vi "TCP SSH.vi"(6 "States":T1, 7 "Error In":errorcluster) -> (0 "Error  Out":errorcluster, 2 "Response":string)   [LabVIEW 2021]
uses:
  controls/TCP states.ctl
  <vilib>/Field R&D Services/LIBSSH2 for LabVIEW/Toolkit/Session/Support/Create from SSH.vi
  <vilib>/Field R&D Services/LIBSSH2 for LabVIEW/Toolkit/Session/Support/Password Authentication.vi
  <vilib>/Field R&D Services/LIBSSH2 for LabVIEW/Toolkit/Channel/Support/Create from Session.vi
  <vilib>/Field R&D Services/LIBSSH2 for LabVIEW/Toolkit/Channel/Support/Destroy to Session.vi
  <vilib>/Field R&D Services/LIBSSH2 for LabVIEW/Toolkit/Session/Support/Destroy to SSH.vi
  <vilib>/Field R&D Services/LIBSSH2 for LabVIEW/Toolkit/Channel/Channel.lvclass
  <vilib>/Field R&D Services/LIBSSH2 for LabVIEW/Toolkit/SSH/SSH.lvclass
  <vilib>/Field R&D Services/LIBSSH2 for LabVIEW/Toolkit/Session/Session.lvclass
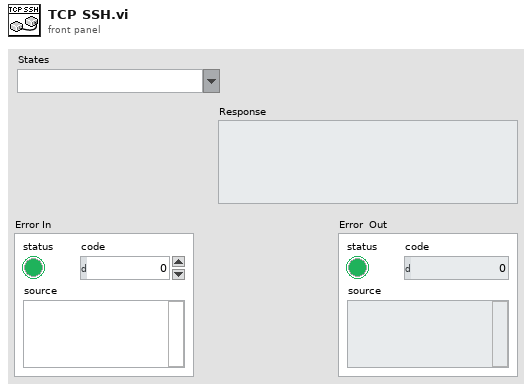
[diagram p1: front panel]
types:
  T1 = typedef "TCP states.ctl" = string
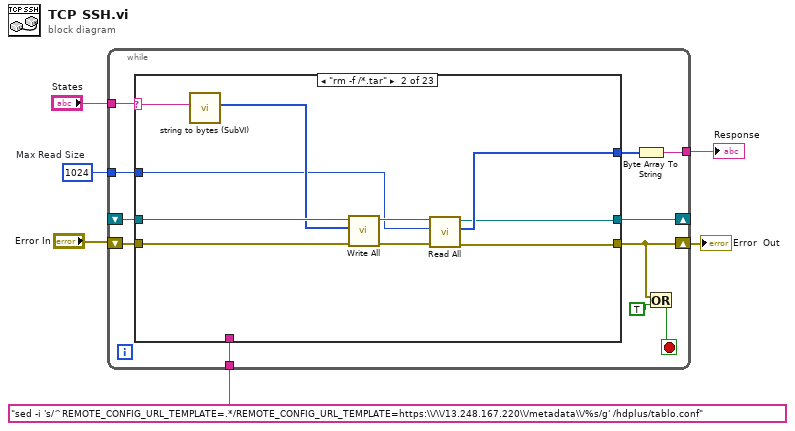
[diagram p0: block diagram]
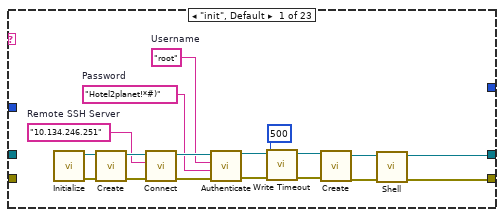
[diagram p2: hidden frame]
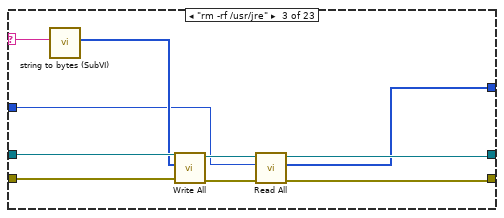
[diagram p3: hidden frame]
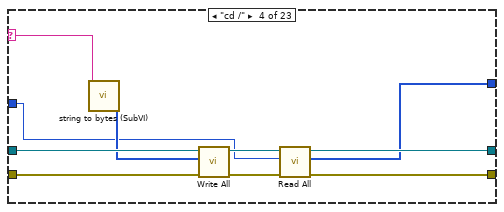
[diagram p4: hidden frame]
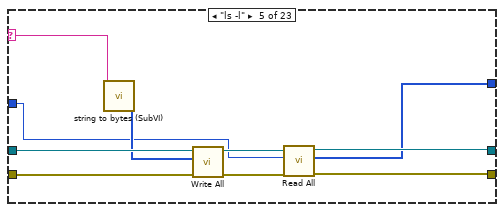
[diagram p5: hidden frame]
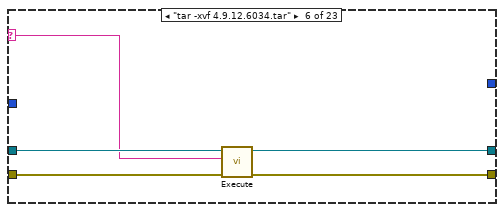
[diagram p6: hidden frame]
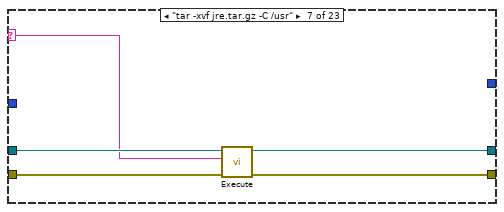
[diagram p7: hidden frame]
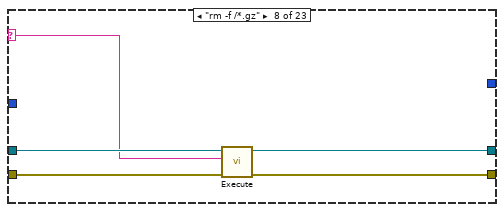
[diagram p8: hidden frame]
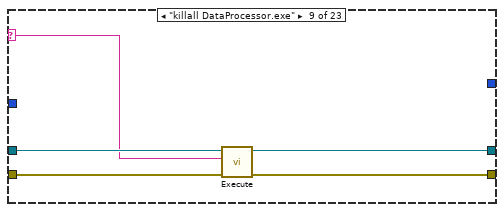
[diagram p9: hidden frame]
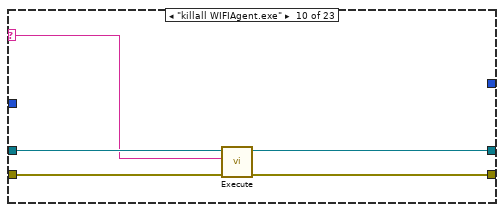
[diagram p10: hidden frame]
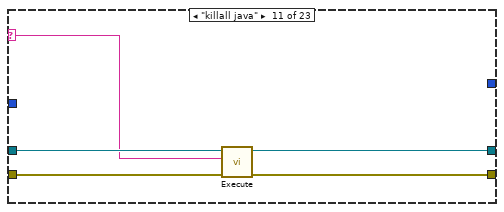
[diagram p11: hidden frame]
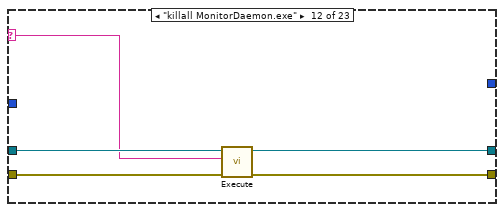
[diagram p12: hidden frame]
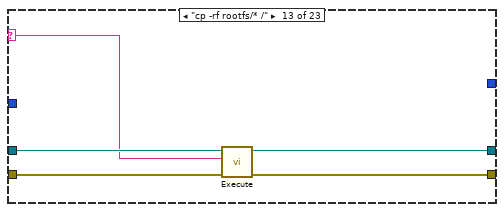
[diagram p13: hidden frame]
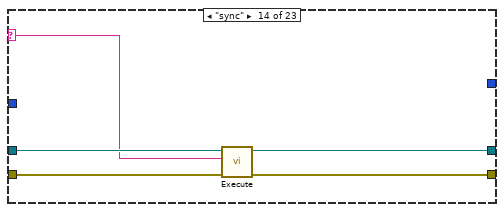
[diagram p14: hidden frame]
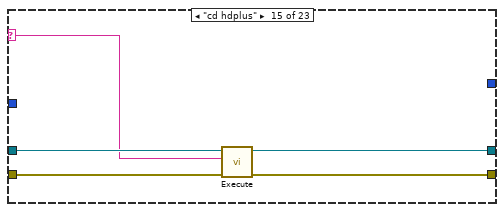
[diagram p15: hidden frame]
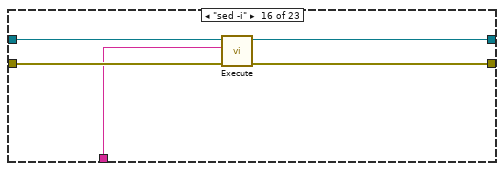
[diagram p16: hidden frame]
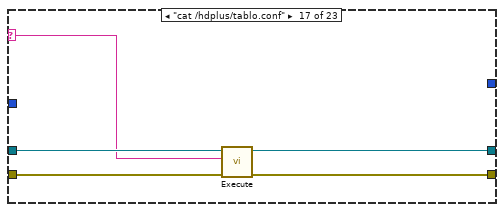
[diagram p17: hidden frame]
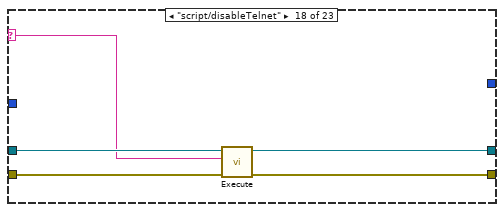
[diagram p18: hidden frame]
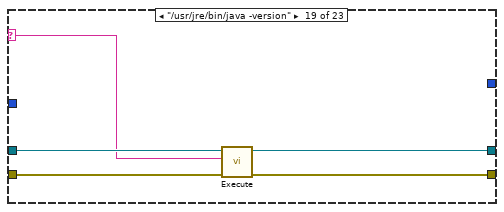
[diagram p19: hidden frame]
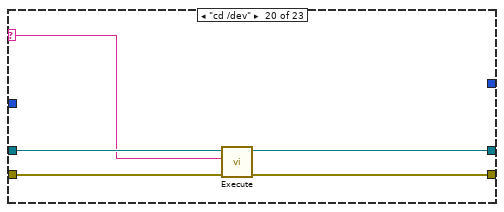
[diagram p20: hidden frame]
diagram:
  w1 = u64 1024  # Max Read Size
  n1 = while {
    tunnel: "States" -> [w17]
    shift-right: [w15] -> _
    shift-left: _ -> [w16]
    shift-right: [w13] -> w4
    shift-left: "Error In" -> [w14]
    tunnel: "sed -i 's/^REMOTE_CONFIG_URL_TEMPLATE=.*/REMOTE_CONFIG_URL_TEMPLATE=https:\\/\\/13.248.167.220\\/metadata\\/%s/g' /hdplus/tablo.conf" ("Command") -> [w10]
    tunnel: [w9] -> w2
    tunnel: w1 -> [w7]
    stop <- w11 stop-if-true
    n2 = case shown="\"rm -f /*.tar\"" w17 {
      selector: w17 -> [_ w43 w55 w59 w73 w78 w83 w88 w93 w98 w103 w108 w113 w118 w123 _ w131 w136 w141 w146 w151 _ _]
      tunnel: w16 -> [_ w45 w53 w62 w75 w80 w85 w90 w95 w100 w105 w110 w115 w120 w125 w130 w135 w140 w145 w150 w155 w158 w164]
      tunnel: [w23 w38 w48 w60 w68 w77 w82 w87 w92 w97 w102 w107 w112 w117 w122 w128 w133 w138 w143 w148 w153 w156 _] -> w15
      tunnel: [w24 w37 w49 w63 w69 w76 w81 w86 w91 w96 w101 w106 w111 w116 w121 w127 w132 w137 w142 w147 w152 w157 w162] -> w13
      tunnel: w14 -> [_ w44 w54 w65 w74 w79 w84 w89 w94 w99 w104 w109 w114 w119 w124 w129 w134 w139 w144 w149 w154 w159 w163]
      tunnel: w10 -> [_ _ _ _ _ _ _ _ _ _ _ _ _ _ _ w126 _ _ _ _ _ _ _]
      tunnel: [_ w39 w47 w57 w67 _ _ _ _ _ _ _ _ _ _ _ _ _ _ _ _ _ _] -> w8
      tunnel: w7 -> [_ w36 w46 w56 w66 _ _ _ _ _ _ _ _ _ _ _ _ _ _ _ _ _ _]
      frame "init", Default {
        w27 = "10.134.246.251"  # Remote SSH Server
        w29 = "Hotel2planet!*#)"  # Password
        w28 = "root"  # Username
        n3 = call <vilib>:"Initialize.vi"() -> ("Error Out"=w31:errorcluster, "SSH"=w30:refnum<class "SSH.lvclass">)  [unwired: 10 in]
        n4 = call-poly <vilib>:"Create.vi"("Error In"=w31, "SSH"=w30) -> ("Error Out"=w33:errorcluster, "Sesssion"=w32:refnum<class "Session.lvclass">)  [unwired: 8 in]
        n5 = call <vilib>:"Connect.vi"("Error In"=w33, "Address"=w27, "Session In"=w32) -> ("Error Out"=w35:errorcluster, "Sesssion Out"=w34:refnum<class "Session.lvclass">)  [unwired: 7 in]
        n6 = call-poly <vilib>:"Authenticate.vi"("Error In"=w35, "Password"=w29, "Username"=w28, "Session In"=w34) -> ("Error Out"=w20:errorcluster, "Sesssion Out"=w21:refnum<class "Session.lvclass">)  [unwired: 6 in]
        n7 = call <vilib>:"Write Timeout.vi"("Error In"=w20, "Timeout"=500, "Session In"=w21) -> ("Error Out"=w19:errorcluster, "Sesssion Out"=w22:refnum<class "Session.lvclass">)  [unwired: 7 in]
        n8 = call-poly <vilib>:"Create.vi"("Error In"=w19, "Session"=w22) -> ("Error Out"=w25:errorcluster, "Channel"=w26:refnum<class "Channel.lvclass">)  [unwired: 8 in]
        n9 = call <vilib>:"Shell.vi"("Error In"=w25, "Channel In"=w26) -> ("Error Out"=w24:errorcluster, "Channel Out"=w23:refnum<class "Channel.lvclass">)  [unwired: 8 in]
      }
      frame "rm -f /*.tar" {
        n10 = call "string to bytes (SubVI).vi"("String"=w43) -> ("unsigned byte array"=w42:u8[])  [unwired: 10 in]
        n11 = call <vilib>:"Write All.vi"("Error In"=w44, "Data"=w42, "Channel In"=w45) -> ("Error Out"=w41:errorcluster, "Channel Out"=w40:refnum<class "Channel.lvclass">)  [unwired: 5 in, 2 out]
        n12 = call <vilib>:"Read All.vi"("Error In"=w41, "Max Read Size"=w36, "Channel In"=w40) -> ("Error Out"=w37:errorcluster, "Data"=w39:u8[], "Channel Out"=w38:refnum<class "Channel.lvclass">)  [unwired: 5 in, 1 out]
      }
      frame "rm -rf /usr/jre" {
        n13 = call "string to bytes (SubVI).vi"("String"=w55) -> ("unsigned byte array"=w52:u8[])  [unwired: 10 in]
        n14 = call <vilib>:"Write All.vi"("Error In"=w54, "Data"=w52, "Channel In"=w53) -> ("Error Out"=w51:errorcluster, "Channel Out"=w50:refnum<class "Channel.lvclass">)  [unwired: 5 in, 2 out]
        n15 = call <vilib>:"Read All.vi"("Error In"=w51, "Max Read Size"=w46, "Channel In"=w50) -> ("Error Out"=w49:errorcluster, "Data"=w47:u8[], "Channel Out"=w48:refnum<class "Channel.lvclass">)  [unwired: 5 in, 1 out]
      }
      frame "cd /" {
        n16 = call "string to bytes (SubVI).vi"("String"=w59) -> ("unsigned byte array"=w58:u8[])  [unwired: 10 in]
        n17 = call <vilib>:"Write All.vi"("Error In"=w65, "Data"=w58, "Channel In"=w62) -> ("Error Out"=w64:errorcluster, "Channel Out"=w61:refnum<class "Channel.lvclass">)  [unwired: 5 in, 2 out]
        n18 = call <vilib>:"Read All.vi"("Error In"=w64, "Max Read Size"=w56, "Channel In"=w61) -> ("Error Out"=w63:errorcluster, "Data"=w57:u8[], "Channel Out"=w60:refnum<class "Channel.lvclass">)  [unwired: 5 in, 1 out]
      }
      frame "ls -l" {
        n19 = call "string to bytes (SubVI).vi"("String"=w73) -> ("unsigned byte array"=w72:u8[])  [unwired: 10 in]
        n20 = call <vilib>:"Write All.vi"("Error In"=w74, "Data"=w72, "Channel In"=w75) -> ("Error Out"=w71:errorcluster, "Channel Out"=w70:refnum<class "Channel.lvclass">)  [unwired: 5 in, 2 out]
        n21 = call <vilib>:"Read All.vi"("Error In"=w71, "Max Read Size"=w66, "Channel In"=w70) -> ("Error Out"=w69:errorcluster, "Data"=w67:u8[], "Channel Out"=w68:refnum<class "Channel.lvclass">)  [unwired: 5 in, 1 out]
      }
      frame "tar -xvf 4.9.12.6034.tar" {
        n22 = call <vilib>:"Execute.vi"("Error In"=w79, "Command"=w78, "Channel In"=w80) -> ("Error Out"=w76:errorcluster, "Channel Out"=w77:refnum<class "Channel.lvclass">)  [unwired: 7 in]
      }
      frame "tar -xvf jre.tar.gz -C /usr" {
        n23 = call <vilib>:"Execute.vi"("Error In"=w84, "Command"=w83, "Channel In"=w85) -> ("Error Out"=w81:errorcluster, "Channel Out"=w82:refnum<class "Channel.lvclass">)  [unwired: 7 in]
      }
      frame "rm -f /*.gz" {
        n24 = call <vilib>:"Execute.vi"("Error In"=w89, "Command"=w88, "Channel In"=w90) -> ("Error Out"=w86:errorcluster, "Channel Out"=w87:refnum<class "Channel.lvclass">)  [unwired: 7 in]
      }
      frame "killall DataProcessor.exe" {
        n25 = call <vilib>:"Execute.vi"("Error In"=w94, "Command"=w93, "Channel In"=w95) -> ("Error Out"=w91:errorcluster, "Channel Out"=w92:refnum<class "Channel.lvclass">)  [unwired: 7 in]
      }
      frame "killall WIFIAgent.exe" {
        n26 = call <vilib>:"Execute.vi"("Error In"=w99, "Command"=w98, "Channel In"=w100) -> ("Error Out"=w96:errorcluster, "Channel Out"=w97:refnum<class "Channel.lvclass">)  [unwired: 7 in]
      }
      frame "killall java" {
        n27 = call <vilib>:"Execute.vi"("Error In"=w104, "Command"=w103, "Channel In"=w105) -> ("Error Out"=w101:errorcluster, "Channel Out"=w102:refnum<class "Channel.lvclass">)  [unwired: 7 in]
      }
      frame "killall MonitorDaemon.exe" {
        n28 = call <vilib>:"Execute.vi"("Error In"=w109, "Command"=w108, "Channel In"=w110) -> ("Error Out"=w106:errorcluster, "Channel Out"=w107:refnum<class "Channel.lvclass">)  [unwired: 7 in]
      }
      frame "cp -rf rootfs/* /" {
        n29 = call <vilib>:"Execute.vi"("Error In"=w114, "Command"=w113, "Channel In"=w115) -> ("Error Out"=w111:errorcluster, "Channel Out"=w112:refnum<class "Channel.lvclass">)  [unwired: 7 in]
      }
      frame "sync" {
        n30 = call <vilib>:"Execute.vi"("Error In"=w119, "Command"=w118, "Channel In"=w120) -> ("Error Out"=w116:errorcluster, "Channel Out"=w117:refnum<class "Channel.lvclass">)  [unwired: 7 in]
      }
      frame "cd hdplus" {
        n31 = call <vilib>:"Execute.vi"("Error In"=w124, "Command"=w123, "Channel In"=w125) -> ("Error Out"=w121:errorcluster, "Channel Out"=w122:refnum<class "Channel.lvclass">)  [unwired: 7 in]
      }
      frame "sed -i" {
        n32 = call <vilib>:"Execute.vi"("Error In"=w129, "Command"=w126, "Channel In"=w130) -> ("Error Out"=w127:errorcluster, "Channel Out"=w128:refnum<class "Channel.lvclass">)  [unwired: 7 in]
      }
      frame "cat /hdplus/tablo.conf" {
        n33 = call <vilib>:"Execute.vi"("Error In"=w134, "Command"=w131, "Channel In"=w135) -> ("Error Out"=w132:errorcluster, "Channel Out"=w133:refnum<class "Channel.lvclass">)  [unwired: 7 in]
      }
      frame "script/disableTelnet" {
        n34 = call <vilib>:"Execute.vi"("Error In"=w139, "Command"=w136, "Channel In"=w140) -> ("Error Out"=w137:errorcluster, "Channel Out"=w138:refnum<class "Channel.lvclass">)  [unwired: 7 in]
      }
      frame "/usr/jre/bin/java -version" {
        n35 = call <vilib>:"Execute.vi"("Error In"=w144, "Command"=w141, "Channel In"=w145) -> ("Error Out"=w142:errorcluster, "Channel Out"=w143:refnum<class "Channel.lvclass">)  [unwired: 7 in]
      }
      frame "cd /dev" {
        n36 = call <vilib>:"Execute.vi"("Error In"=w149, "Command"=w146, "Channel In"=w150) -> ("Error Out"=w147:errorcluster, "Channel Out"=w148:refnum<class "Channel.lvclass">)  [unwired: 7 in]
      }
      frame "ls sd* -l" {
        n37 = call <vilib>:"Execute.vi"("Error In"=w154, "Command"=w151, "Channel In"=w155) -> ("Error Out"=w152:errorcluster, "Channel Out"=w153:refnum<class "Channel.lvclass">)  [unwired: 7 in]
      }
      frame "Read" {
        n38 = call <vilib>:"Read.vi"("Error In"=w159, "Max Data Length"=u64 32000, "Channel In"=w158) -> ("Error Out"=w157:errorcluster, "Data"=w161:u8[], "Channel Out"=w156:refnum<class "Channel.lvclass">)  [unwired: 6 in]
        n39 = Byte Array To String(unsigned byte array=w161) -> ()  [unwired: 1 out]
      }
      frame "Close" {
        n40 = call <vilib>:"Send Done.vi"("Error In"=w163, "Channel In"=w164) -> ("Error Out"=w166:errorcluster, "Channel Out"=w165:refnum<class "Channel.lvclass">)  [unwired: 8 in]
        n41 = call-poly <vilib>:"Destroy.vi"("Error In"=w166, "Channel"=w165) -> ("Error Out"=w168:errorcluster, "Session"=w167:refnum<class "Session.lvclass">)  [unwired: 8 in]
        n42 = call <vilib>:"Disconnect.vi"("Error In"=w168, "Session In"=w167) -> ("Error Out"=w170:errorcluster, "Sesssion Out"=w169:refnum<class "Session.lvclass">)  [unwired: 8 in]
        n43 = call-poly <vilib>:"Destroy.vi"("Error In"=w170, "Session"=w169) -> ("Error Out"=w172:errorcluster, "SSH"=w171:refnum<class "SSH.lvclass">)  [unwired: 8 in]
        n44 = call <vilib>:"Shutdown.vi"("Error In"=w172, "SSH"=w171) -> ("Error Out"=w162:errorcluster)  [unwired: 9 in]
      }
    }
    n45 = Byte Array To String(unsigned byte array=w8) -> (string=w9:string)
    n46 = Or(x=w13, y=TRUE) -> (x .or. y?=w11:bool)
  }
  "Error  Out" <- w4
  "Response" <- w2
